vi "Engine - Initialize HW.vi"(8 "error in (no error)":errorcluster, 10 "DMM-Switch Configuration":T1={"DMM Resource Name"="", "DMM Measurement"=enum."DC Volts", "DMM Resolution in Digits"=0.0, "DMM Range [EU]"=0.0, "DMM Temp - Value"={"DMM Temp - Transducer Type"=1, "DMM Temp - Thermocouple Type"=6, "DMM Temp - Fixed Reference Junction"=25.0, "DMM Temp - RTD Type"=enum."Pt3851", "DMM Temp - RTD Resistance"=100.0, "DMM Temp - Thermistor Type"=enum."44006", "DMM Temp - RTD A"=0.0039083, "DMM Temp - RTD B"=-5.775e-07, "DMM Temp - RTD C"=-4.183e-12, "DMM Temp - Thermistor A"=0.0010295, "DMM Temp - Thermistor B"=0.0002391, "DMM Temp - Thermistor C"=1.568e-07}, "Switch Resource Name"="", "Switch Topology"="", "Switch Scan List"="", "Switch Trigger Source"=enum."Immediate", "Switch Scan Advanced Output"=enum."None", "DMM Measurement Complete"=enum."None", "DMM Trigger Source"=enum."Immediate", "# of Channels"=0, "Group CH Names - Configuration"="", "Group CH Names - Input Channels"="", "Group CH Names - Measurement Channels"="", "Group CH Names - Runtime Status"=""} {"DMM Temp - Value"."DMM Temp - Thermistor C" format="%#_13g"; "DMM Temp - Value"."DMM Temp - Thermistor B" format="%#_13g"; "DMM Temp - Value"."DMM Temp - Thermistor A" format="%#_13g"; "DMM Temp - Value"."DMM Temp - RTD Resistance" format="%.2f"; "DMM Temp - Value"."DMM Temp - Fixed Reference Junction" format="%.2f"; "DMM Temp - Value"."DMM Temp - Thermocouple Type" items=["B"=1, "E"=4, "J"=6, "K"=7, "N"=8, "R"=9, "S"=10, "T"=11]; "DMM Temp - Value"."DMM Temp - Transducer Type" items=["Thermocouple"=1, "Thermistor"=2, "2-Wire RTD"=3, "4-Wire RTD"=4]; "DMM Resolution in Digits" items=["3 1/2"=3.5, "4 1/2"=4.5, "5 1/2"=5.5, "6 1/2"=6.5, "7 1/2"=7.5]}) -> (0 "error out":errorcluster, 2 "DMM Ref Out":refnum<k15>, 3 "Switch Ref Out":refnum<k15>)   [LabVIEW 2016, in "DMM-SWITCH-ScanList Engine.lvlib"]
doc: "Initialize and configure Switch and DMM devices for a Hardware Triggered Scan List Measurement configured with the parameters coming from the DMM-Switch Configuration Cluster."
uses:
  DMM-SWITCH-ScanList Engine.lvlib
  TypeDefs/DMM-Switch Configuration.ctl
  <instrlib>/niDMM/nidmm.llb/niDMM Function.ctl
  <instrlib>/niDMM/nidmm.llb/niDMM Resolution in Digits.ctl
  System Explorer/Pages/Configuration Controls/DMM Temp.ctl
  <instrlib>/niDMM/nidmm.llb/niDMM Transducer Type.ctl
  <instrlib>/niDMM/nidmm.llb/niDMM Thermocouple Type.ctl
  <instrlib>/niDMM/nidmm.llb/niDMM RTD Type.ctl
  <instrlib>/niDMM/nidmm.llb/niDMM Thermistor Type.ctl
  <instrlib>/niSwitch/niSwitch.llb/niSwitch Topologies.ctl
  <instrlib>/niSwitch/niSwitch.llb/niSwitch Trigger Input.ctl
  <instrlib>/niSwitch/niSwitch.llb/niSwitch Scan Advanced Output.ctl
  <instrlib>/niDMM/nidmm.llb/niDMM Measurement Complete.ctl
  <instrlib>/niDMM/nidmm.llb/niDMM Trigger.ctl
  <instrlib>/niDMM/nidmm.llb/niDMM Sample Trigger.ctl
  <instrlib>/niDMM/nidmm.llb/niDMM Reference Junction Type.ctl
  <instrlib>/niDMM/nidmm.llb/niDMM Configure Measurement Digits.vi
  System Explorer/DMM-SWITCH-ScanList System Explorer.lvlib
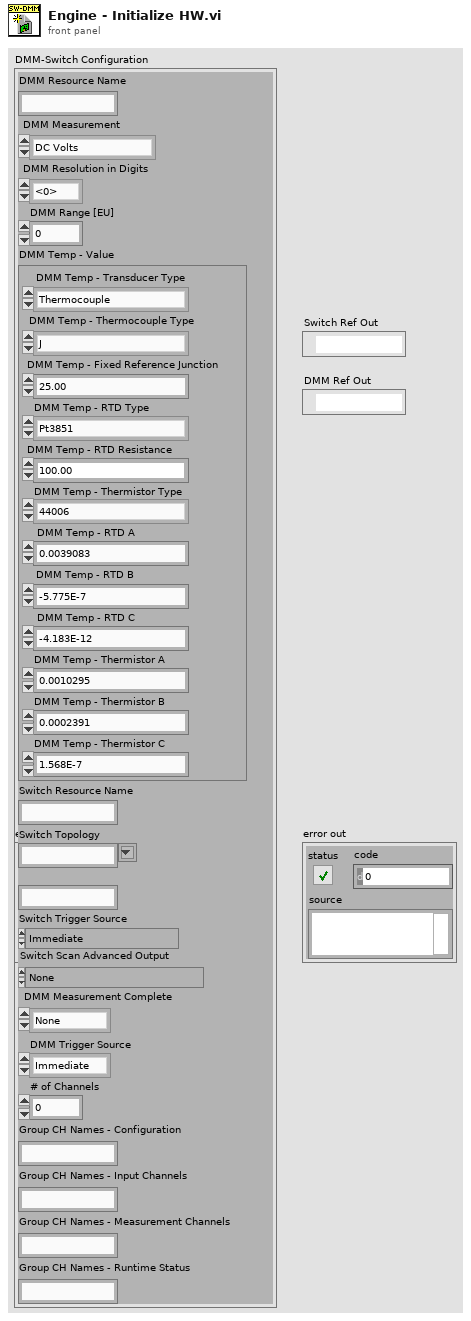
[diagram p1: front panel]
types:
  T1 = typedef "DMM-SWITCH-ScanList Engine.lvlib/DMM-Switch Configuration.ctl" = cluster{"DMM Resource Name":string, "DMM Measurement":T2, "DMM Resolution in Digits":T3, "DMM Range [EU]":dbl, "DMM Temp - Value":T4, "Switch Resource Name":string, "Switch Topology":T9, "Switch Scan List":string, "Switch Trigger Source":T10, "Switch Scan Advanced Output":T11, "DMM Measurement Complete":T12, "DMM Trigger Source":T13, "# of Channels":u32, "Group CH Names - Configuration":string, "Group CH Names - Input Channels":string, "Group CH Names - Measurement Channels":string, "Group CH Names - Runtime Status":string}
  T2 = typedef "niDMM Function.ctl" = enum16{"DC Volts", "AC Volts", "DC Current", "AC Current", "2-wire Resistance", "4-wire Resistance", "Diode", "Frequency", "Period", "AC Volts DC Coupled", "Capacitance", "Inductance", "Temperature"}
  T3 = typedef "niDMM Resolution in Digits.ctl" = dbl
  T4 = typedef "DMM-SWITCH-ScanList System Explorer.lvlib/DMM Temp.ctl" = cluster{"DMM Temp - Transducer Type":T5, "DMM Temp - Thermocouple Type":T6, "DMM Temp - Fixed Reference Junction":dbl, "DMM Temp - RTD Type":T7, "DMM Temp - RTD Resistance":dbl, "DMM Temp - Thermistor Type":T8, "DMM Temp - RTD A":dbl, "DMM Temp - RTD B":dbl, "DMM Temp - RTD C":dbl, "DMM Temp - Thermistor A":dbl, "DMM Temp - Thermistor B":dbl, "DMM Temp - Thermistor C":dbl}
  T5 = typedef "niDMM Transducer Type.ctl" = i32
  T6 = typedef "niDMM Thermocouple Type.ctl" = i32
  T7 = typedef "niDMM RTD Type.ctl" = enum16{"Custom", "Pt3750", "Pt3851", "Pt3911", "Pt3916", "Pt3920", "Pt3928"}
  T8 = typedef "niDMM Thermistor Type.ctl" = enum16{"Custom", "44004", "44006", "44007"}
  T9 = typedef "niSwitch Topologies.ctl" = string
  T10 = typedef "niSwitch Trigger Input.ctl" = enum16{"Immediate", "External", "TTL0", "TTL1", "TTL2", "TTL3", "TTL4", "TTL5", "TTL6", "TTL7", "ECL0", "ECL1", "PXI Star", "Software Trigger Function", "Rear Connector", "Front Connector", "Rear Connector of Module 1", "Rear Connector of Module 2", "Rear Connector of Module 3", "Rear Connector of Module 4", "Rear Connector of Module 5", "Rear Connector of Module 6", "Rear Connector of Module 7", "Rear Connector of Module 8", "Rear Connector of Module 9", "Rear Connector of Module 10", "Rear Connector of Module 11", "Rear Connector of Module 12", "Front Connector of Module 1", "Front Connector of Module 2", "Front Connector of Module 3", "Front Connector of Module 4", "Front Connector of Module 5", "Front Connector of Module 6", "Front Connector of Module 7", "Front Connector of Module 8", "Front Connector of Module 9", "Front Connector of Module 10", "Front Connector of Module 11", "Front Connector of Module 12"}
  T11 = typedef "niSwitch Scan Advanced Output.ctl" = enum16{"None", "External", "TTL0", "TTL1", "TTL2", "TTL3", "TTL4", "TTL5", "TTL6", "TTL7", "ECL0", "ECL1", "PXI Star", "Rear Connector", "Front Connector", "Rear Connector Module 1", "Rear Connector Module 2", "Rear Connector Module 3", "Rear Connector Module 4", "Rear Connector Module 5", "Rear Connector Module 6", "Rear Connector Module 7", "Rear Connector Module 8", "Rear Connector Module 9", "Rear Connector Module 10", "Rear Connector Module 11", "Rear Connector Module 12", "Front Connector Module 1", "Front Connector Module 2", "Front Connector Module 3", "Front Connector Module 4", "Front Connector Module 5", "Front Connector Module 6", "Front Connector Module 7", "Front Connector Module 8", "Front Connector Module 9", "Front Connector Module 10", "Front Connector Module 11", "Front Connector Module 12"}
  T12 = typedef "niDMM Measurement Complete.ctl" = enum16{"None", "External", "TTL 0", "TTL 1", "TTL 2", "TTL 3", "TTL 4", "TTL 5", "TTL 6", "TTL 7", "LBR Trig 0"}
  T13 = typedef "niDMM Trigger.ctl" = enum16{"Immediate", "External", "TTL 0", "TTL 1", "TTL 2", "TTL 3", "TTL 4", "TTL 5", "TTL 6", "Software", "TTL 7", "PXI Star", "LBR Trig 1", "Aux Trig 1"}
  T14 = typedef "niDMM Sample Trigger.ctl" = enum16{"Immediate", "External", "TTL 0", "TTL 1", "TTL 2", "TTL 3", "TTL 4", "TTL 5", "TTL 6", "Interval", "Software", "TTL 7", "PXI Star", "LBR Trig 1", "Aux Trig 1"}
  T15 = typedef "niDMM Reference Junction Type.ctl" = i32
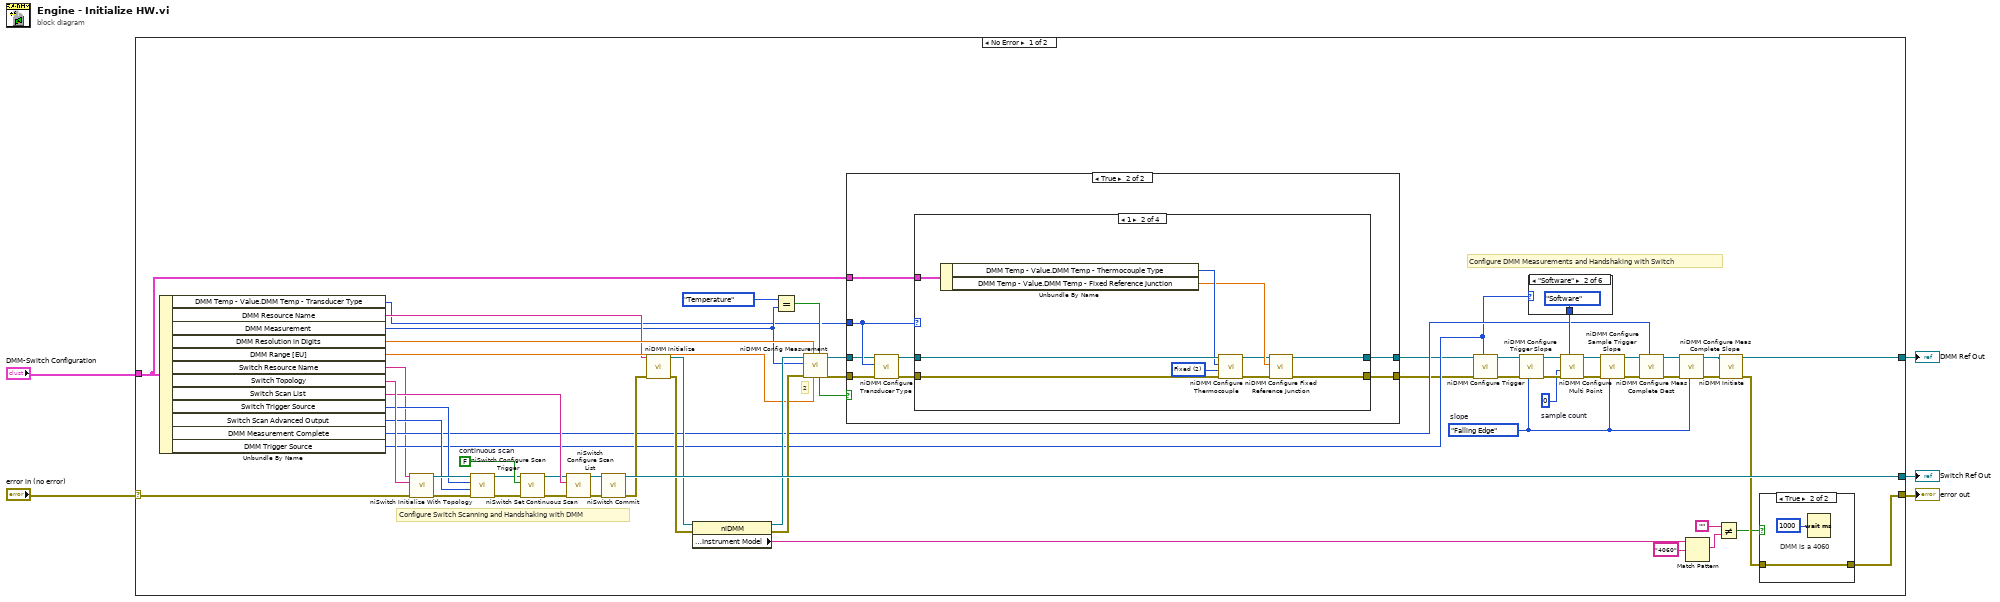
[diagram p0: block diagram]
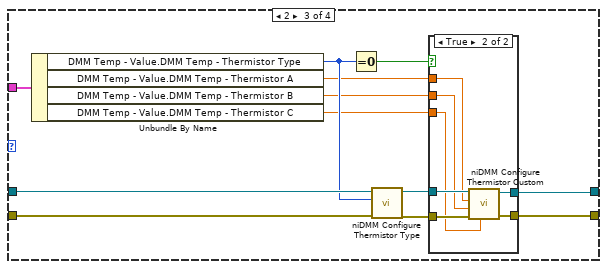
[diagram p4: hidden frame]
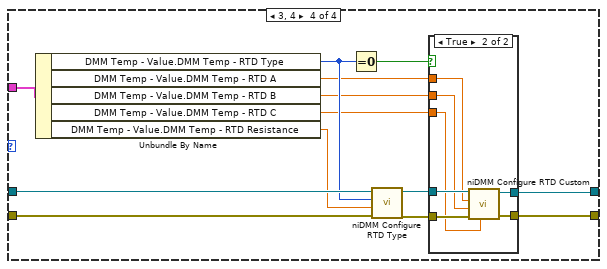
[diagram p6: hidden frame]
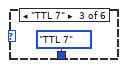
[diagram p10: hidden frame]
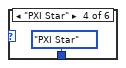
[diagram p11: hidden frame]
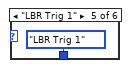
[diagram p12: hidden frame]
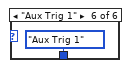
[diagram p13: hidden frame]
diagram:
  n1 = case shown="No Error" "error in (no error)" {
    selector: "error in (no error)" -> [w27 w138]
    tunnel: [w63 _] -> w5
    tunnel: [w62 w138] -> w4
    tunnel: [w61 _] -> w3
    tunnel: "DMM-Switch Configuration" -> [w10 _]
    frame No Error {
      w41 = enum16{"Rising Edge", "Falling Edge"}."Falling Edge"  # slope
      w52 = 0  # sample count
      w34 = FALSE  # continuous scan
      # "Configure DMM Measurements and Handshaking with Switch"
      # "Configure Switch Scanning and Handshaking with DMM"
      # "2"
      n2 = Unbundle By Name(w10) -> ("DMM Temp - Value.DMM Temp - Transducer Type"=w11:T5, "DMM Resource Name"=w17:string, "DMM Measurement"=w13:T2, "DMM Resolution in Digits"=w23:T3, "DMM Range [EU]"=w22:dbl, "Switch Resource Name"=w15:string, "Switch Topology"=w37:T9, "Switch Scan List"=w35:string, "Switch Trigger Source"=w21:T10, "Switch Scan Advanced Output"=w20:T11, "DMM Measurement Complete"=w19:T12, "DMM Trigger Source"=w18:T13)
      n3 = call <instrlib>:"niSwitch Initialize With Topology.vi"("error in (no error)"=w27, "topology name"=w37, "resource name"=w15) -> ("error out"=w16:errorcluster, "instrument handle out"=w32:refnum<k15>)  [unwired: 2 in, 5 out]
      n4 = call <instrlib>:"niSwitch Configure Scan Trigger.vi"("error in (no error)"=w16, "scan advanced output (External)"=w20, "trigger input (External)"=w21, "instrument handle"=w32) -> ("error out"=w36:errorcluster, "instrument handle out"=w33:refnum<k15>)  [unwired: 1 in, 5 out]
      n5 = call <instrlib>:"niSwitch Set Continuous Scan.vi"("error in (no error)"=w36, "continuous scan (False)"=w34, "instrument handle"=w33) -> ("error out"=w26:errorcluster, "instrument handle out"=w31:refnum<k15>)  [unwired: 7 out]
      n6 = call <instrlib>:"niSwitch Configure Scan List.vi"("error in (no error)"=w26, "scan list"=w35, "instrument handle"=w31) -> ("error out"=w25:errorcluster, "instrument handle out"=w30:refnum<k15>)  [unwired: 1 in, 6 out]
      n7 = call <instrlib>:"niSwitch Commit.vi"("error in (no error)"=w25, "instrument handle"=w30) -> ("error out"=w24:errorcluster, "instrument handle out"=w63:refnum<k15>)  [unwired: 8 out]
      n8 = call <instrlib>:"niDMM Initialize.vi"("error in (no error)"=w24, "Instrument Descriptor"=w17) -> ("error out"=w28:errorcluster, "instrument handle out"=w39:refnum<k15>)  [unwired: 2 in, 6 out]
      n9 = property class="niDMM"(reference=w39, error in=w28) -> (reference out=w38:refnum<k15>, error out=w29:errorcluster, "Inherent IVI Attributes:Instrument Identification:Instrument Model"=w40:string)
      n10 = Equal?(x=niDMM_Function."Temperature" ("DMM Measurement"), y=w13) -> (x = y?=w12:bool)
      n11 = call-poly <instrlib>:"niDMM Config Measurement.vi"("Range"=w22, "Resolution in Digits"=w23, "error in (no error)"=w29, "Function"=w13, "instrument handle"=w38) -> ("error out"=w9:errorcluster, "instrument handle out"=w8:refnum<k15>)  [unwired: 5 out]
      n12 = case shown="True" w12 {
        tunnel: w11 -> [_ w73]
        tunnel: w10 -> [_ w71]
        tunnel: w9 -> [w64 w69]
        tunnel: w8 -> [w65 w68]
        tunnel: [w65 w67] -> w6
        tunnel: [w64 w66] -> w7
        frame False {
        }
        frame True {
          n13 = call <instrlib>:"niDMM Configure Transducer Type.vi"("error in (no error)"=w69, "Transducer Type"=w73, "instrument handle"=w68) -> ("error out"=w70:errorcluster, "instrument handle out"=w72:refnum<k15>)  [unwired: 7 in]
          n14 = case shown="1" w73 {
            tunnel: w72 -> [w75 w85 w95 w117]
            tunnel: w71 -> [_ w84 w97 w119]
            tunnel: w70 -> [w74 w78 w96 w118]
            tunnel: [w75 w77 w91 w113] -> w67
            tunnel: [w74 w76 w90 w112] -> w66
            frame 0, Default {
            }
            frame 1 {
              w82 = T15 2 items=["Fixed"=2] ("Reference Junction Type")
              n15 = Unbundle By Name(w84) -> ("DMM Temp - Value.DMM Temp - Thermocouple Type"=w83:T6, "DMM Temp - Value.DMM Temp - Fixed Reference Junction"=w81:dbl)
              n16 = call <instrlib>:"niDMM Configure Thermocouple.vi"("error in (no error)"=w78, "Reference Junction Type"=w82, "Thermocouple Type"=w83, "instrument handle"=w85) -> ("error out"=w79:errorcluster, "instrument handle out"=w80:refnum<k15>)  [unwired: 6 in]
              n17 = call <instrlib>:"niDMM Configure Fixed Reference Junction.vi"("error in (no error)"=w79, "Fixed Reference Junction"=w81, "instrument handle"=w80) -> ("error out"=w76:errorcluster, "instrument handle out"=w77:refnum<k15>)  [unwired: 7 in]
            }
            frame 2 {
              n18 = Unbundle By Name(w97) -> ("DMM Temp - Value.DMM Temp - Thermistor Type"=w94:T8, "DMM Temp - Value.DMM Temp - Thermistor A"=w88:dbl, "DMM Temp - Value.DMM Temp - Thermistor B"=w87:dbl, "DMM Temp - Value.DMM Temp - Thermistor C"=w86:dbl)
              n19 = Equal To 0?(x=w94) -> (x = 0?=w93:bool)
              n20 = call <instrlib>:"niDMM Configure Thermistor Type.vi"("error in (no error)"=w96, "Thermistor Type"=w94, "instrument handle"=w95) -> ("error out"=w89:errorcluster, "instrument handle out"=w92:refnum<k15>)  [unwired: 7 in]
              n21 = case shown="True" w93 {
                tunnel: w92 -> [w99 w106]
                tunnel: [w99 w105] -> w91
                tunnel: [w98 w104] -> w90
                tunnel: w89 -> [w98 w103]
                tunnel: w88 -> [_ w102]
                tunnel: w87 -> [_ w101]
                tunnel: w86 -> [_ w100]
                frame False {
                }
                frame True {
                  n22 = call <instrlib>:"niDMM Configure Thermistor Custom.vi"("C"=w100, "error in (no error)"=w103, "B"=w101, "A"=w102, "instrument handle"=w106) -> ("error out"=w104:errorcluster, "instrument handle out"=w105:refnum<k15>)  [unwired: 5 in]
                }
              }
            }
            frame 3, 4 {
              n23 = Unbundle By Name(w119) -> ("DMM Temp - Value.DMM Temp - RTD Type"=w116:T7, "DMM Temp - Value.DMM Temp - RTD A"=w110:dbl, "DMM Temp - Value.DMM Temp - RTD B"=w109:dbl, "DMM Temp - Value.DMM Temp - RTD C"=w108:dbl, "DMM Temp - Value.DMM Temp - RTD Resistance"=w107:dbl)
              n24 = Equal To 0?(x=w116) -> (x = 0?=w115:bool)
              n25 = call <instrlib>:"niDMM Configure RTD Type.vi"("error in (no error)"=w118, "RTD Resistance"=w107, "RTD Type"=w116, "instrument handle"=w117) -> ("error out"=w111:errorcluster, "instrument handle out"=w114:refnum<k15>)  [unwired: 6 in]
              n26 = case shown="True" w115 {
                tunnel: w114 -> [w121 w128]
                tunnel: [w121 w127] -> w113
                tunnel: [w120 w126] -> w112
                tunnel: w111 -> [w120 w125]
                tunnel: w110 -> [_ w124]
                tunnel: w109 -> [_ w123]
                tunnel: w108 -> [_ w122]
                frame False {
                }
                frame True {
                  n27 = call <instrlib>:"niDMM Configure RTD Custom.vi"("C"=w122, "error in (no error)"=w125, "B"=w123, "A"=w124, "instrument handle"=w128) -> ("error out"=w126:errorcluster, "instrument handle out"=w127:refnum<k15>)  [unwired: 5 in]
                }
              }
            }
          }
        }
      }
      n28 = call <instrlib>:"niDMM Configure Trigger.vi"("Trigger Source"=w18, "error in (no error)"=w7, "instrument handle"=w6) -> ("error out"=w57:errorcluster, "instrument handle out"=w58:refnum<k15>)  [unwired: 1 in, 6 out]
      n29 = call <instrlib>:"niDMM Configure Trigger Slope.vi"("Slope"=w41, "error in (no error)"=w57, "instrument handle"=w58) -> ("error out"=w55:errorcluster, "instrument handle out"=w56:refnum<k15>)  [unwired: 7 out]
      n30 = case shown="\"Software\"" w18 {
        selector: w18 -> [w132 _ _ _ _ _]
        tunnel: [w132 niDMM_Sample_Trigger."Software" ("Sample Trigger") niDMM_Sample_Trigger."TTL 7" ("Sample Trigger") niDMM_Sample_Trigger."PXI Star" ("Sample Trigger") niDMM_Sample_Trigger."LBR Trig 1" ("Sample Trigger") niDMM_Sample_Trigger."Aux Trig 1" ("Sample Trigger")] -> w51
        frame "Immediate", Default {
        }
        frame "Software" {
        }
        frame "TTL 7" {
        }
        frame "PXI Star" {
        }
        frame "LBR Trig 1" {
        }
        frame "Aux Trig 1" {
        }
      }
      n31 = call <instrlib>:"niDMM Configure Multi Point.vi"("Sample Trigger"=w51, "error in (no error)"=w55, "Sample Count"=w52, "instrument handle"=w56) -> ("error out"=w53:errorcluster, "instrument handle out"=w54:refnum<k15>)  [unwired: 2 in, 4 out]
      n32 = call <instrlib>:"niDMM Configure Sample Trigger Slope.vi"("Slope"=w41, "error in (no error)"=w53, "instrument handle"=w54) -> ("error out"=w47:errorcluster, "instrument handle out"=w46:refnum<k15>)  [unwired: 7 out]
      n33 = call <instrlib>:"niDMM Configure Meas Complete Dest.vi"("Measurement Complete Destination"=w19, "error in (no error)"=w47, "instrument handle"=w46) -> ("error out"=w42:errorcluster, "instrument handle out"=w45:refnum<k15>)  [unwired: 7 out]
      n34 = call <instrlib>:"niDMM Configure Meas Complete Slope.vi"("Slope"=w41, "error in (no error)"=w42, "instrument handle"=w45) -> ("error out"=w43:errorcluster, "instrument handle out"=w44:refnum<k15>)  [unwired: 7 out]
      n35 = Match Pattern(string=w40, regular expression="4060") -> (match substring=w49:string)  [unwired: 4 out]
      n36 = Not Equal?(x="", y=w49) -> (x != y?=w59:bool)
      n37 = call <instrlib>:"niDMM Initiate.vi"("error in (no error)"=w43, "instrument handle"=w44) -> ("error out"=w60:errorcluster, "instrument handle out"=w61:refnum<k15>)  [unwired: 8 out]
      n38 = case shown="True" w59 {
        tunnel: w60 -> [w129 w130]
        tunnel: [w129 w130] -> w62
        frame False {
          # "DMM is \nnot a 4060"
        }
        frame True {
          # "DMM is a 4060"
          n39 = Wait (ms)(milliseconds to wait=u32 1000 ("millisecond multiple")) -> ()  [unwired: 1 out]
        }
      }
    }
    frame Error {
    }
  }
  "Switch Ref Out" <- w5
  "error out" <- w4
  "DMM Ref Out" <- w3
